vi "Read instrumentName.vi"(8 "error in (no error)":errorcluster, 11 "instrumentSelect in":refnum<class "InstrumentSelect.lvclass">) -> (0 "error out":errorcluster, 2 "instrumentName":string, 3 "instrumentSelect out":refnum<class "InstrumentSelect.lvclass">)   [LabVIEW 2014, in "TCSDataDefinitions.lvlib" / "TCSCommand.lvlib" / "InstrumentSelect.lvclass"]
uses:
  InstrumentSelect.lvclass
  InstrumentSelect.lvclass/InstrumentSelect.ctl
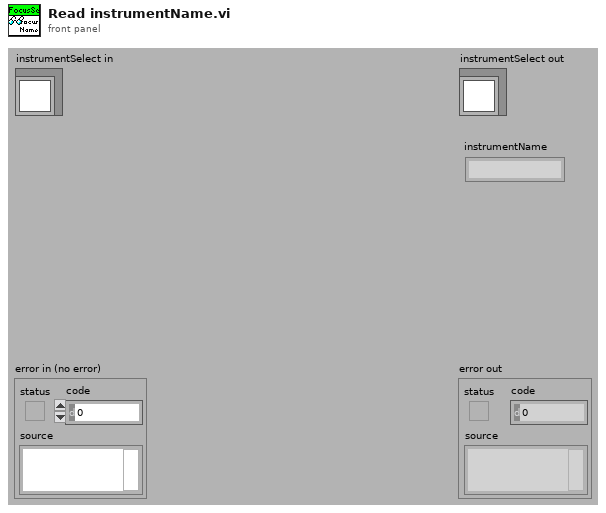
[diagram p1: front panel]
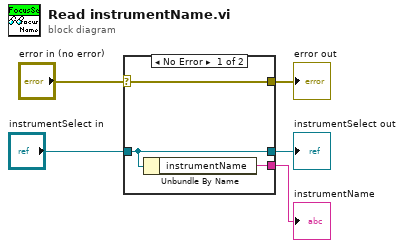
[diagram p0: block diagram]
diagram:
  n1 = case shown="No Error" "error in (no error)" {
    selector: "error in (no error)" -> [w8 w9]
    tunnel: [w8 w9] -> w4
    tunnel: [w7 w10] -> w2
    tunnel: "instrumentSelect in" -> [w7 w10]
    tunnel: [w6 _] -> w1
    frame No Error {
      n2 = Unbundle By Name(w7) -> ("instrumentName"=w6:string)
    }
    frame Error {
    }
  }
  "error out" <- w4
  "instrumentSelect out" <- w2
  "instrumentName" <- w1
